vi "Read Write Default Parameters.vi"(0 "Default Parameters":T1, 11 "Error in (no error)":errorcluster, 13 "Operations":enum16{"Read Parameters", "Write Parameters"}(ring)=enum."Write Parameters") -> (4 "Default Parameters Our":T1, 15 "Error out":errorcluster)   [LabVIEW 2022 SP3]
uses:
  <vilib>/Utility/config.llb/NI_LVConfig.lvlib
  <vilib>/Utility/config.llb/Write Key (Boolean).vi
  <vilib>/Utility/config.llb/Read Key (Boolean).vi
  <vilib>/Utility/config.llb/Read Key (Double).vi
  <vilib>/Utility/config.llb/Write Key (Double).vi
  <vilib>/Utility/config.llb/Read Key (U32).vi
  <vilib>/Utility/config.llb/Read Key (String).vi
  <vilib>/Utility/config.llb/Write Key (U32).vi
  Controls/Parameter Settings.ctl
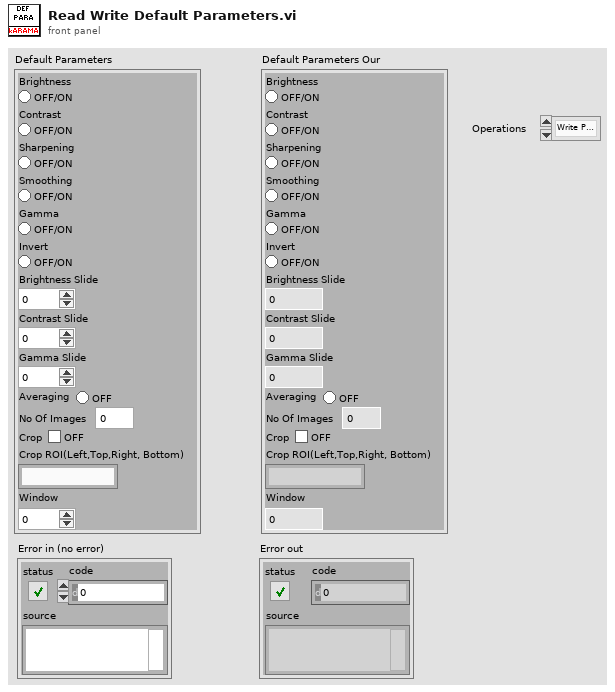
[diagram p1: front panel]
types:
  T1 = typedef "Parameter Settings.ctl" = cluster{"Brightness":bool, "Contrast":bool, "Sharpening":bool, "Smoothing":bool, "Gamma":bool, "Invert":bool, "Brightness Slide":dbl, "Contrast Slide":dbl, "Gamma Slide":dbl, "Averaging":bool, "No Of Images":u32, "Crop":bool, "Crop ROI(Left,Top,Right, Bottom)":string, "Window":u32}
  T2 = typedef "Paths.ctl" = cluster{"Configuration":path, "Event Logs":path, "Error Logs":path, "Configuration.ini":path}
  T3 = typedef "NI_LVConfig.lvlib/Config Data RefNum.ctl" = refnum<k1>
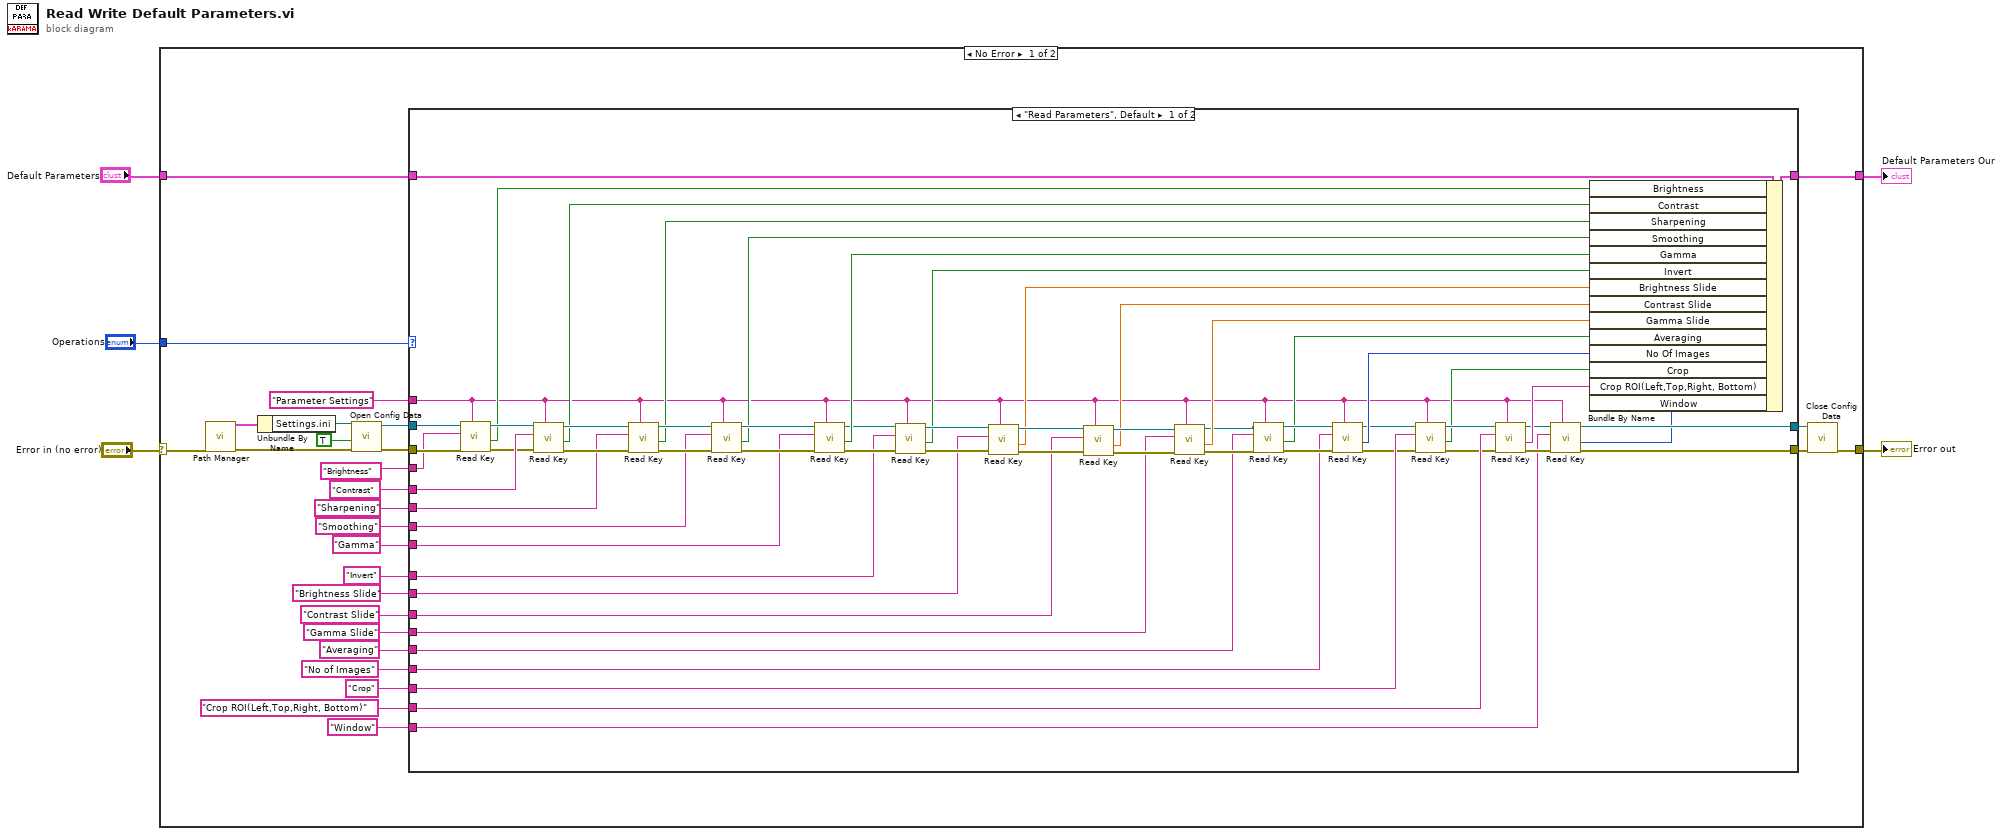
[diagram p0: block diagram]
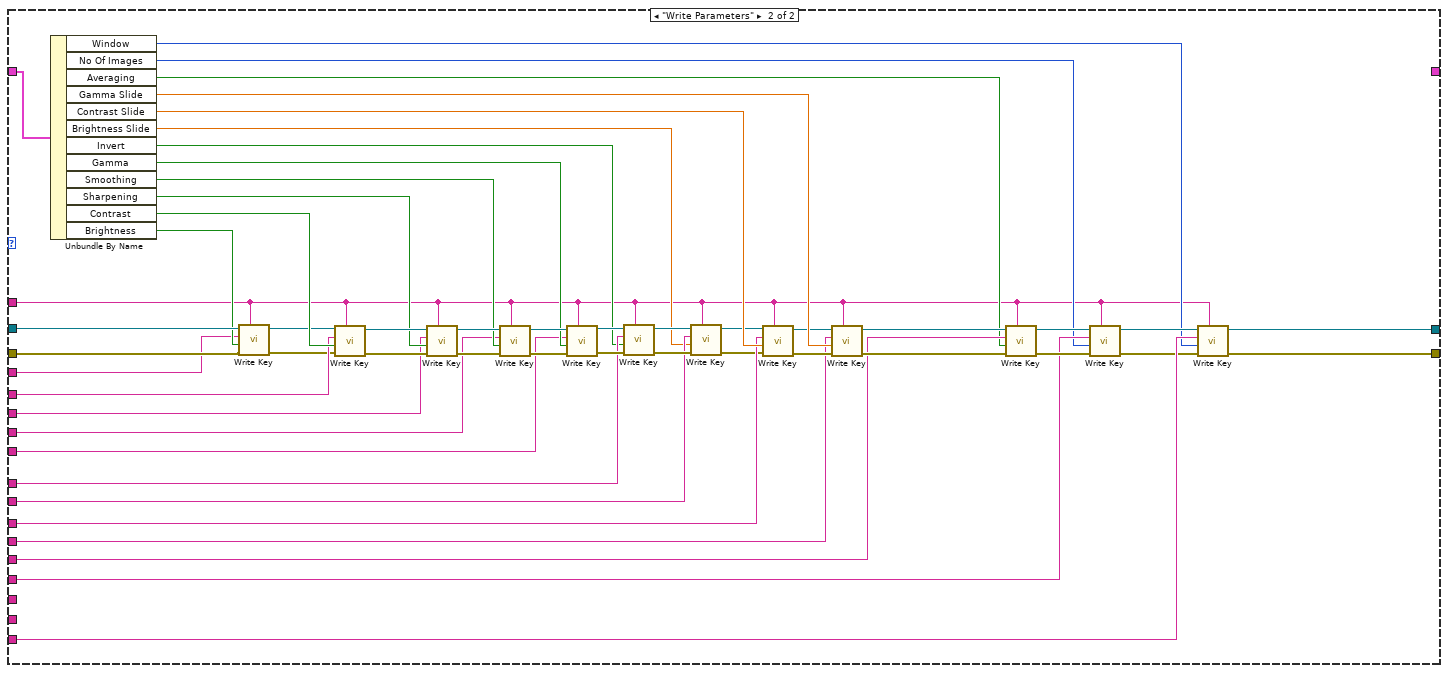
[diagram p2: hidden frame]
diagram:
  n1 = case shown="No Error" "Error in (no error)" {
    selector: "Error in (no error)" -> [w33 w147]
    tunnel: [w32 w147] -> w4
    tunnel: "Operations" -> [w31 _]
    tunnel: "Default Parameters" -> [w30 _]
    tunnel: [w29 _] -> w1
    frame No Error {
      n2 = call "Path Manager.vi"("error in (no error)"=w33) -> ("Cluster"=w28:T2, "Error out"=w27:errorcluster)  [unwired: 13 in]
      n3 = Unbundle By Name(w28) -> ("Settings.ini"=w24:path)
      n4 = call <vilib>:"Open Config Data.vi"("error in (no error)"=w27, "create file if necessary (T)"=TRUE, "configuration file path"=w24) -> ("error out"=w26:errorcluster, "refnum"=w23:T3)  [unwired: 6 in, 1 out]
      n5 = case shown="\"Read Parameters\", Default" w31 {
        tunnel: [w37 w96] -> w25
        tunnel: w30 -> [w84 w146]
        tunnel: w26 -> [w68 w115]
        tunnel: w23 -> [w70 w113]
        tunnel: [w39 w100] -> w22
        tunnel: "Gamma Slide" ("key") -> [w62 w131]
        tunnel: "Contrast Slide" ("key") -> [w63 w130]
        tunnel: "Gamma" ("key") -> [w88 w129]
        tunnel: "Smoothing" ("key") -> [w89 w128]
        tunnel: "Sharpening" ("key") -> [w90 w127]
        tunnel: "Contrast" ("key") -> [w94 w126]
        tunnel: "Parameter Settings" ("section") -> [w34 w95]
        tunnel: [w79 _] -> w29
        tunnel: "Invert" ("key") -> [w65 w119]
        tunnel: "Brightness Slide" ("key") -> [w64 w118]
        tunnel: "Brightness" ("key") -> [w66 w110]
        tunnel: "Averaging" ("key") -> [w51 w105]
        tunnel: "No of Images" ("key") -> [w52 w104]
        tunnel: "Crop ROI(Left,Top,Right, Bottom)" ("key") -> [w48 _]
        tunnel: "Crop" ("key") -> [w47 _]
        tunnel: "Window" ("key") -> [w36 w99]
        frame "Read Parameters", Default {
          n6 = call-poly <vilib>:"Read Key.vi"("section"=w34, "error in (no error)"=w68, "key"=w66, "refnum"=w70) -> ("error out"=w67:errorcluster, "value"=w61:bool, "refnum out"=w69:T3)  [unwired: 4 in, 1 out]
          n7 = call-poly <vilib>:"Read Key.vi"("section"=w34, "error in (no error)"=w67, "key"=w94, "refnum"=w69) -> ("error out"=w93:errorcluster, "value"=w80:bool, "refnum out"=w85:T3)  [unwired: 4 in, 1 out]
          n8 = call-poly <vilib>:"Read Key.vi"("section"=w34, "error in (no error)"=w93, "key"=w90, "refnum"=w85) -> ("error out"=w92:errorcluster, "value"=w81:bool, "refnum out"=w86:T3)  [unwired: 4 in, 1 out]
          n9 = call-poly <vilib>:"Read Key.vi"("section"=w34, "error in (no error)"=w92, "key"=w89, "refnum"=w86) -> ("error out"=w91:errorcluster, "value"=w82:bool, "refnum out"=w87:T3)  [unwired: 4 in, 1 out]
          n10 = call-poly <vilib>:"Read Key.vi"("section"=w34, "error in (no error)"=w91, "key"=w88, "refnum"=w87) -> ("error out"=w74:errorcluster, "value"=w83:bool, "refnum out"=w78:T3)  [unwired: 4 in, 1 out]
          n11 = call-poly <vilib>:"Read Key.vi"("section"=w34, "error in (no error)"=w74, "key"=w65, "refnum"=w78) -> ("error out"=w73:errorcluster, "value"=w60:bool, "refnum out"=w77:T3)  [unwired: 4 in, 1 out]
          n12 = call-poly <vilib>:"Read Key.vi"("section"=w34, "error in (no error)"=w73, "key"=w64, "refnum"=w77) -> ("error out"=w72:errorcluster, "value"=w59:dbl, "refnum out"=w76:T3)  [unwired: 4 in, 1 out]
          n13 = call-poly <vilib>:"Read Key.vi"("section"=w34, "error in (no error)"=w72, "key"=w63, "refnum"=w76) -> ("error out"=w71:errorcluster, "value"=w58:dbl, "refnum out"=w75:T3)  [unwired: 4 in, 1 out]
          n14 = call-poly <vilib>:"Read Key.vi"("section"=w34, "error in (no error)"=w71, "key"=w62, "refnum"=w75) -> ("error out"=w54:errorcluster, "value"=w57:dbl, "refnum out"=w56:T3)  [unwired: 4 in, 1 out]
          n15 = call-poly <vilib>:"Read Key.vi"("section"=w34, "error in (no error)"=w54, "key"=w51, "refnum"=w56) -> ("error out"=w53:errorcluster, "value"=w50:bool, "refnum out"=w55:T3)  [unwired: 4 in, 1 out]
          n16 = call-poly <vilib>:"Read Key.vi"("section"=w34, "error in (no error)"=w53, "key"=w52, "refnum"=w55) -> ("error out"=w46:errorcluster, "value"=w49:u32, "refnum out"=w44:T3)  [unwired: 4 in, 1 out]
          n17 = call-poly <vilib>:"Read Key.vi"("section"=w34, "error in (no error)"=w46, "key"=w47, "refnum"=w44) -> ("error out"=w45:errorcluster, "value"=w42:bool, "refnum out"=w43:T3)  [unwired: 4 in, 1 out]
          n18 = call-poly <vilib>:"Read Key.vi"("section"=w34, "error in (no error)"=w45, "key"=w48, "refnum"=w43) -> ("error out"=w38:errorcluster, "value"=w41:string, "refnum out"=w40:T3)  [unwired: 4 in, 1 out]
          n19 = call-poly <vilib>:"Read Key.vi"("section"=w34, "error in (no error)"=w38, "key"=w36, "refnum"=w40) -> ("error out"=w37:errorcluster, "value"=w35:u32, "refnum out"=w39:T3)  [unwired: 4 in, 1 out]
          n20 = Bundle By Name(cluster=w84, "Brightness"=w61, "Contrast"=w80, "Sharpening"=w81, "Smoothing"=w82, "Gamma"=w83, "Invert"=w60, "Brightness Slide"=w59, "Contrast Slide"=w58, "Gamma Slide"=w57, "Averaging"=w50, "No Of Images"=w49, "Crop"=w42, "Crop ROI(Left,Top,Right, Bottom)"=w41, "Window"=w35) -> (w79:T1)
        }
        frame "Write Parameters" {
          n21 = Unbundle By Name(w146) -> ("Window"=w98:u32, "No Of Images"=w102:u32, "Averaging"=w103:bool, "Gamma Slide"=w139:dbl, "Contrast Slide"=w140:dbl, "Brightness Slide"=w116:dbl, "Invert"=w117:bool, "Gamma"=w132:bool, "Smoothing"=w133:bool, "Sharpening"=w134:bool, "Contrast"=w135:bool, "Brightness"=w111:bool)
          n22 = call-poly <vilib>:"Write Key.vi"("section"=w95, "error in (no error)"=w115, "value"=w111, "key"=w110, "refnum"=w113) -> ("error out"=w114:errorcluster, "refnum out"=w112:T3)  [unwired: 4 in, 1 out]
          n23 = call-poly <vilib>:"Write Key.vi"("section"=w95, "error in (no error)"=w114, "value"=w135, "key"=w126, "refnum"=w112) -> ("error out"=w144:errorcluster, "refnum out"=w145:T3)  [unwired: 4 in, 1 out]
          n24 = call-poly <vilib>:"Write Key.vi"("section"=w95, "error in (no error)"=w144, "value"=w134, "key"=w127, "refnum"=w145) -> ("error out"=w143:errorcluster, "refnum out"=w136:T3)  [unwired: 4 in, 1 out]
          n25 = call-poly <vilib>:"Write Key.vi"("section"=w95, "error in (no error)"=w143, "value"=w133, "key"=w128, "refnum"=w136) -> ("error out"=w142:errorcluster, "refnum out"=w137:T3)  [unwired: 4 in, 1 out]
          n26 = call-poly <vilib>:"Write Key.vi"("section"=w95, "error in (no error)"=w142, "value"=w132, "key"=w129, "refnum"=w137) -> ("error out"=w120:errorcluster, "refnum out"=w123:T3)  [unwired: 4 in, 1 out]
          n27 = call-poly <vilib>:"Write Key.vi"("section"=w95, "error in (no error)"=w120, "value"=w117, "key"=w119, "refnum"=w123) -> ("error out"=w124:errorcluster, "refnum out"=w125:T3)  [unwired: 4 in, 1 out]
          n28 = call-poly <vilib>:"Write Key.vi"("section"=w95, "error in (no error)"=w124, "value"=w116, "key"=w118, "refnum"=w125) -> ("error out"=w121:errorcluster, "refnum out"=w122:T3)  [unwired: 4 in, 1 out]
          n29 = call-poly <vilib>:"Write Key.vi"("section"=w95, "error in (no error)"=w121, "value"=w140, "key"=w130, "refnum"=w122) -> ("error out"=w141:errorcluster, "refnum out"=w138:T3)  [unwired: 4 in, 1 out]
          n30 = call-poly <vilib>:"Write Key.vi"("section"=w95, "error in (no error)"=w141, "value"=w139, "key"=w131, "refnum"=w138) -> ("error out"=w106:errorcluster, "refnum out"=w109:T3)  [unwired: 4 in, 1 out]
          n31 = call-poly <vilib>:"Write Key.vi"("section"=w95, "error in (no error)"=w106, "value"=w103, "key"=w105, "refnum"=w109) -> ("error out"=w107:errorcluster, "refnum out"=w108:T3)  [unwired: 4 in, 1 out]
          n32 = call-poly <vilib>:"Write Key.vi"("section"=w95, "error in (no error)"=w107, "value"=w102, "key"=w104, "refnum"=w108) -> ("error out"=w97:errorcluster, "refnum out"=w101:T3)  [unwired: 4 in, 1 out]
          n33 = call-poly <vilib>:"Write Key.vi"("section"=w95, "error in (no error)"=w97, "value"=w98, "key"=w99, "refnum"=w101) -> ("error out"=w96:errorcluster, "refnum out"=w100:T3)  [unwired: 4 in, 1 out]
        }
      }
      n34 = call <vilib>:"Close Config Data.vi"("error in (no error)"=w25, "refnum"=w22) -> ("error out"=w32:errorcluster)  [unwired: 8 in, 1 out]
    }
    frame Error {
    }
  }
  "Error out" <- w4
  "Default Parameters Our" <- w1
